vi "Tear Down.vi"(8 "error in (no error)":errorcluster, 11 "Car Position Simulator in":refnum<class "Car Position Simulator.lvclass">) -> (0 "error out":errorcluster, 3 "Car Position Simulator out":refnum<class "Car Position Simulator.lvclass">)   [LabVIEW 2016, in "CLD Exam - Car Wash.lvlib" / "Car Position Simulator.lvclass"]
uses:
  Car Position Simulator.lvclass
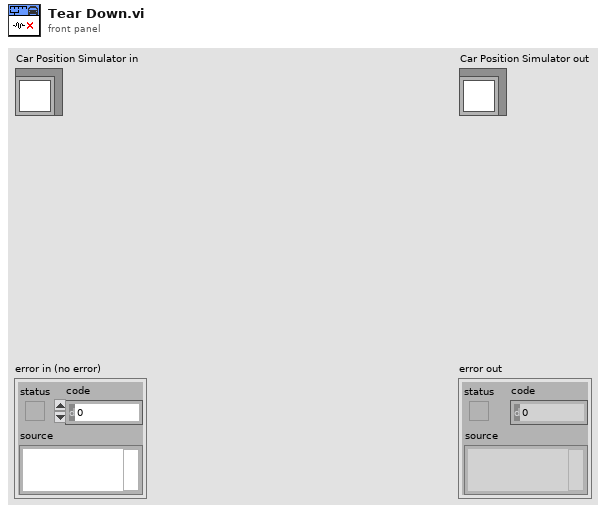
[diagram p1: front panel]
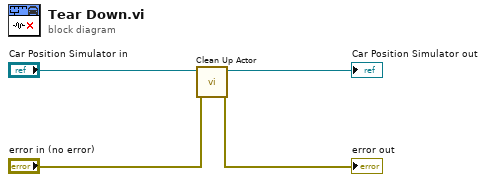
[diagram p0: block diagram]
diagram:
  n1 = call-dynamic "Clean Up Actor.vi"("error in (no error)"="error in (no error)", "Car Position Simulator in"="Car Position Simulator in") -> ("error out"=→"error out":errorcluster, "Car Position Simulator out"=→"Car Position Simulator out":refnum<class "Car Position Simulator.lvclass">)  [unwired: 8 in]
